vi "IsShootToGoal.vi"(0 "object in":refnum<class "DefendAreaTactic.lvclass">, 2 "Ball":refnum<class "Ball.lvclass">, 3 "Field":refnum<class "Field.lvclass">, 5 "error in (no error)":errorcluster) -> (14 "object out":refnum<class "DefendAreaTactic.lvclass">, 16 "IsShoot":bool, 17 "shotTarget":dbl, 19 "error out":errorcluster)   [LabVIEW 2024, in "DefendAreaTactic.lvclass"]
uses:
  DefendAreaTactic.lvclass
  Ball_class/Ball.lvclass
  C:/Users/ROBOIME2/Documents/SSL ROBOIME/SSL_AI/Object_class/Object.lvclass
  Field_class/Field.lvclass
  Object_class/Object.lvclass/Object.ctl
  Ball_class/Ball.lvclass/Ball.ctl
  Field_class/Field.lvclass/Field.ctl
  Object_class/Read x.vi
  Object_class/Read y.vi
  Ball_class/Read v_x.vi
  Ball_class/Read v_y.vi
  Field_class/Read ourGoalPosition.vi
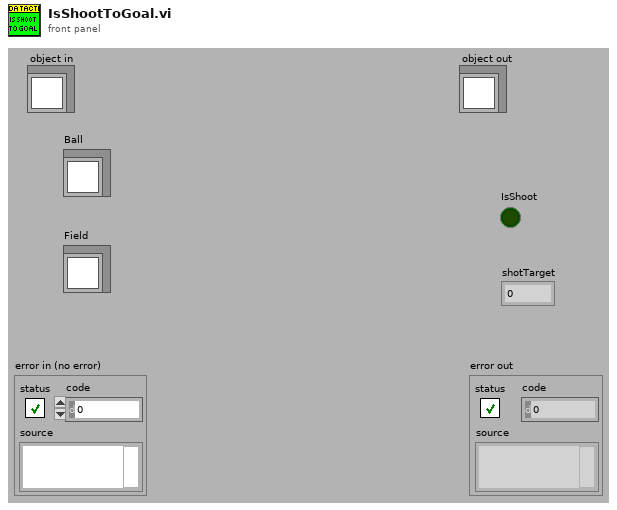
[diagram p1: front panel]
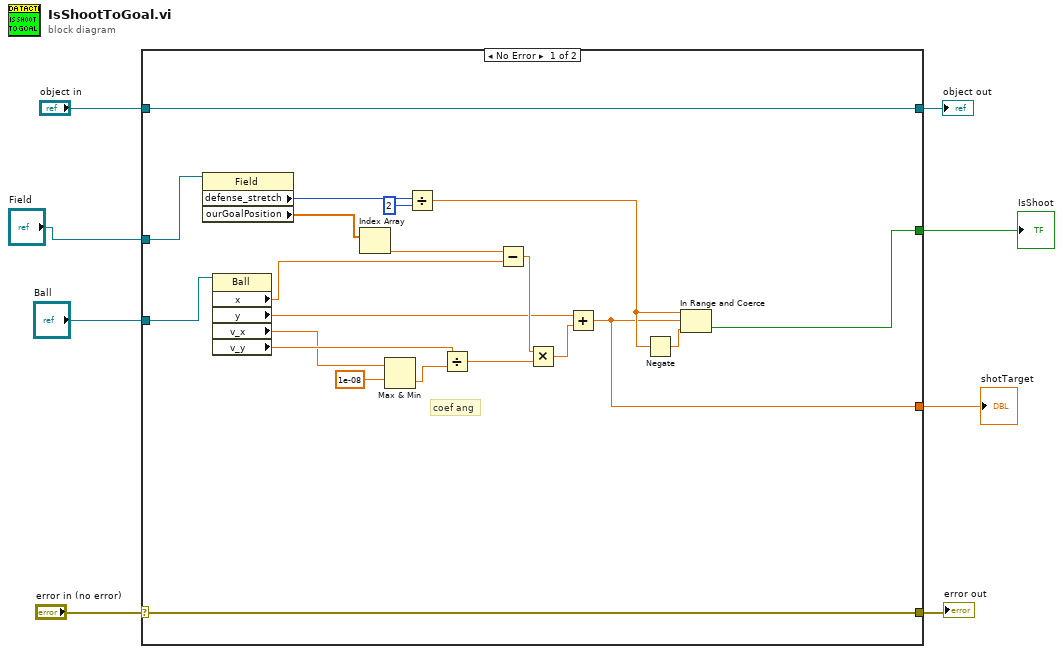
[diagram p0: block diagram]
diagram:
  n1 = case shown="No Error" "error in (no error)" {
    selector: "error in (no error)" -> [w28 w31]
    tunnel: [w28 w31] -> w7
    tunnel: [w29 w30] -> w5
    tunnel: "object in" -> [w29 w30]
    tunnel: "Field" -> [w27 _]
    tunnel: "Ball" -> [w26 _]
    tunnel: [w10 _] -> w2
    tunnel: [w9 _] -> w1
    frame No Error {
      # "coef ang"
      n2 = property class="Field"(reference=w27) -> ("defense_stretch"=w14:i32, "ourGoalPosition"=w21:dbl[])  [unwired: 1 in, 2 out]
      n3 = property class="Ball"(reference=w26) -> ("x"=w17:dbl, "y"=w16:dbl, "v_x"=w23:dbl, "v_y"=w25:dbl)  [unwired: 1 in, 2 out]
      n4 = Index Array(array=w21) -> (element=w20:dbl)  [unwired: 1 in]
      n5 = Max & Min(x=w23, y=1e-08 ("t")) -> (min(x,y)=w22:dbl)  [unwired: 1 out]
      n6 = Divide(x=w14, y=2) -> (x/y=w12:dbl)
      n7 = Divide(x=w25, y=w22) -> (x/y=w18:dbl)
      n8 = Subtract(x=w20, y=w17) -> (x-y=w19:dbl)
      n9 = Multiply(x=w19, y=w18) -> (x*y=w15:dbl)
      n10 = Add(x=w16, y=w15) -> (x+y=w9:dbl)
      n11 = Negate(x=w12) -> (-x=w11:dbl)
      n12 = In Range and Coerce(upper limit=w12, x=w9, lower limit=w11) -> (In Range?=w10:bool)  [unwired: 1 out]
    }
    frame Error {
    }
  }
  "error out" <- w7
  "object out" <- w5
  "IsShoot" <- w2
  "shotTarget" <- w1
